vi "SaveAs.vi"(11 "PluginIniFilePath":path) -> (3 "PluginIniFilePath":path)   [LabVIEW 2018, in "DigitizerPlugins.lvlib"]
uses:
  DigitizerPlugins.lvlib
  <vilib>/Utility/config.llb/NI_LVConfig.lvlib
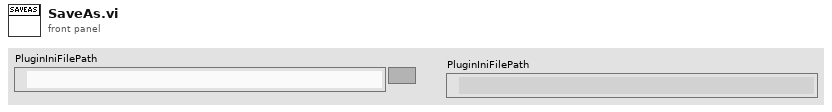
[diagram p1: front panel]
types:
  T1 = typedef "NI_LVConfig.lvlib/Config Data RefNum.ctl" = refnum<k1>
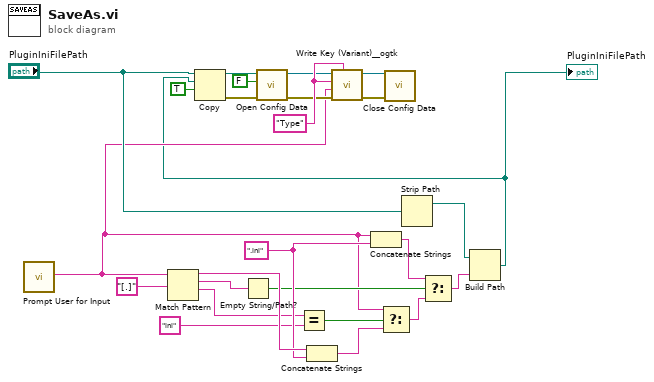
[diagram p0: block diagram]
diagram:
  w10 = "Type" ("key (optional)")
  w23 = ".ini" ("string")
  n1 = call "Prompt User for Input"() -> ("File Name"=w2:string)  [unwired: 16 in, 3 out]
  n2 = Match Pattern(string=w2, regular expression="[.]" ("string")) -> (before substring=w24:string, match substring=w20:string, after substring=w21:string)  [unwired: 1 in, 1 out]
  n3 = Empty String/Path?(string/path=w20) -> (empty?=w15:bool)
  n4 = Equal?(x=w21, y="ini" ("string")) -> (x = y?=w17:bool)
  n5 = Concatenate Strings(w24, w23) -> (w25:string)
  n6 = Concatenate Strings(w2, w23) -> (w16:string)
  n7 = Select(t=w2, s=w17, f=w25) -> (s? t:f=w18:string)
  n8 = Strip Path(path="PluginIniFilePath") -> (stripped path=w13:path)  [unwired: 1 out]
  n9 = Select(t=w16, s=w15, f=w18) -> (s? t:f=w14:string)
  n10 = Build Path(base path=w13, name or relative path=w14) -> (appended path=w1:path)
  "PluginIniFilePath" <- w1
  n11 = Copy(9:TRUE ("overwrite (F)"), 10:w1, 11:"PluginIniFilePath") -> (0:w7:errorcluster, 3:w6:path)  [unwired: 2 in, 1 out]
  n12 = call <vilib>:"Open Config Data.vi"("error in (no error)"=w7, "create file if necessary (T)"=FALSE, "configuration file path"=w6) -> ("error out"=w8:errorcluster, "refnum"=w9:T1)  [unwired: 6 in, 1 out]
  n13 = call <userlib>:"Write Key (Variant)__ogtk.vi"("section"=w10, "error in (no error)"=w8, "key-value"=w2, "key (optional)"=w10, "refnum"=w9) -> ("error out"=w12:errorcluster, "refnum out"=w11:T1)  [unwired: 5 in]
  n14 = call <vilib>:"Close Config Data.vi"("error in (no error)"=w12, "refnum"=w11) -> ()  [unwired: 8 in, 2 out]
